vi "Qtegra_SetMagnet_and_GetData.vi"() -> ()   [LabVIEW 2015]
panel:
  in  "Command2":string="SetIntegrationTime 1.048576"
  in  "Command1":string="SetMagnetDAC 0.3934"
  out "Waveform Chart":dbl(graph)
  out "data of detector":string
  in  "Command3":string="GetData"
  in  "detector":string="H1_CDD"
  out "answer":string
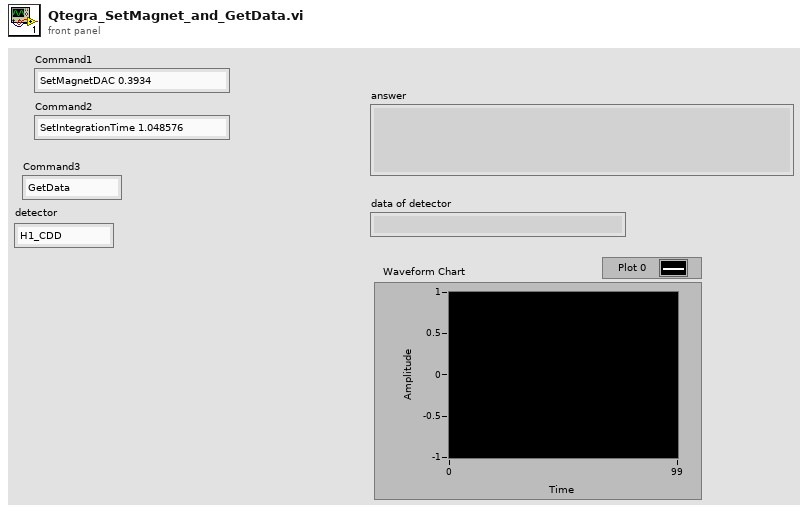
[diagram p1: front panel]
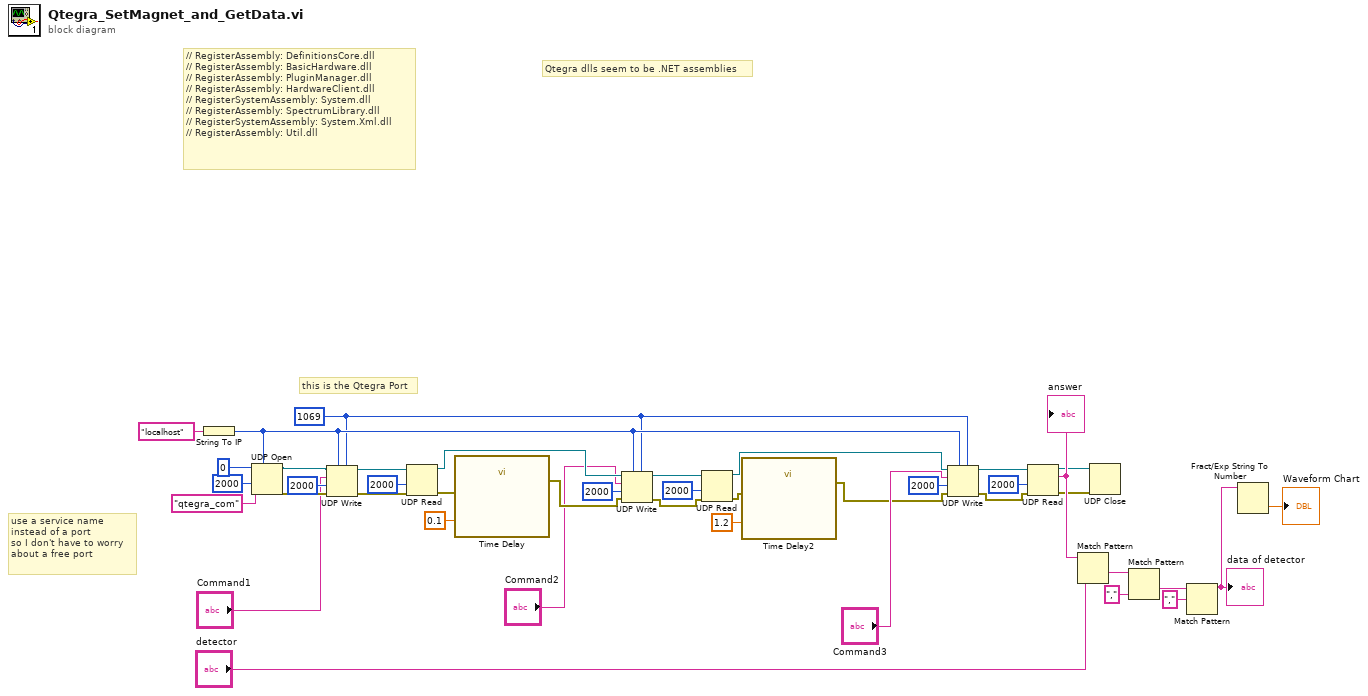
[diagram p0: block diagram]
diagram:
  w1 = u16 1069 ("port or service name")
  # "use a service name\ninstead of a port\nso I don't have to worry\nabout a free port"
  # "this is the Qtegra Port"
  # "Qtegra dlls seem to be .NET assemblies"
  # "// RegisterAssembly: DefinitionsCore.dll\n// RegisterAssembly: BasicHardware.dll\n// RegisterAssembly: PluginManager.dll\n// RegisterAssembly: HardwareClient.dll\n// RegisterSystemAssembly: System.dll\n// RegisterAssembly: SpectrumLibrary.dll\n// RegisterSystemAssembly: System.Xml.dll\n// RegisterAssembly: Util.dll"
  n1 = String To IP(1:"localhost" ("name")) -> (0:w2:u32)
  n2 = UDP Open(7:w2, 9:2000 ("timeout ms (25000)"), 10:"qtegra_com" ("service name"), 11:u16 0 ("port")) -> (port=w38:refnum<k16>, 0:w37:errorcluster)  [unwired: 1 in, 1 out]
  n3 = UDP Write(address=w2, port or service name=w1, connection ID=w38, data in="Command1", 8:w37, 9:2000 ("timeout ms (25000)")) -> (error out=w35:errorcluster, 3:w36:refnum<k16>)
  n4 = UDP Read(connection ID=w36, timeout ms (25000)=2000, 8:w35) -> (error out=w15:errorcluster, 3:w5:refnum<k16>)  [unwired: 1 in, 3 out]
  n5 = call "Time Delay"("error in (no error)"=w15, "Delay Time (s)"=0.1) -> ("error out"=w9:errorcluster)  [unwired: 9 in]
  n6 = UDP Write(address=w2, port or service name=w1, connection ID=w5, data in="Command2", 8:w9, 9:2000 ("timeout ms (25000)")) -> (error out=w13:errorcluster, 3:w12:refnum<k16>)
  n7 = UDP Read(connection ID=w12, timeout ms (25000)=2000, 8:w13) -> (error out=w8:errorcluster, 3:w6:refnum<k16>)  [unwired: 1 in, 3 out]
  n8 = call "Time Delay2"("error in (no error)"=w8, "Delay Time (s)"=1.2) -> ("error out"=w3:errorcluster)  [unwired: 9 in]
  n9 = UDP Write(address=w2, port or service name=w1, connection ID=w6, data in="Command3", 8:w3, 9:2000 ("timeout ms (25000)")) -> (error out=w20:errorcluster, 3:w21:refnum<k16>)
  n10 = UDP Read(connection ID=w21, timeout ms (25000)=2000, 8:w20) -> (data out=w19:string, error out=w17:errorcluster, 3:w18:refnum<k16>)  [unwired: 1 in, 2 out]
  "answer" <- w19
  n11 = Match Pattern(string=w19, regular expression="detector") -> (after substring=w30:string)  [unwired: 1 in, 3 out]
  n12 = UDP Close(connection ID=w18, 8:w17) -> ()  [unwired: 2 out]
  n13 = Match Pattern(string=w30, regular expression=",") -> (after substring=w28:string)  [unwired: 1 in, 3 out]
  n14 = Match Pattern(string=w28, regular expression=",") -> (before substring=w25:string)  [unwired: 1 in, 3 out]
  "data of detector" <- w25
  n15 = Fract/Exp String To Number(string=w25) -> (number=→"Waveform Chart":dbl)  [unwired: 3 in, 1 out]
